vi "Fetch (Waveform).vi"(0 "VISA resource name":refnum<visa-resource-name>, 1 "Segment Index (0)":i32 format="%.0g", 5 "Measurement Source (1: Channel 1)":i32(ring)=1 items=["Channel 1"=1, "Channel 2"=2, "Channel 3"=3, "Channel 4"=4, "Function 1"=5, "Function 2"=6, "Function 3"=7, "Function 4"=8, "Memory 1"=9, "Memory 2"=10, "Memory 3"=11, "Memory 4"=12], 9 "Maximum Time (10000ms)":u32=10000, 11 "error in (no error)":errorcluster) -> (4 "VISA resource name out":refnum<visa-resource-name>, 8 "Waveform Data":waveform(dbl)(graph), 15 "error out":errorcluster)   [LabVIEW 2020, in "Agilent 90000 Series.lvlib"]
doc: "Returns the waveform the oscilloscope acquired for the specified channel. The waveform is from an acquisition that you initiate prior to calling this VI.\n\nYou use the Initiate VI to start an acquisition on the channels that you enable with the Configure Channel VI. The oscilloscope acquires waveforms for the enabled channels concurrently. You must call this VI separately for each enabled channel to obtain the waveforms.\n\nYou can call the Read Waveform VI instead of using low-level VIs.\n\n<B>Note:</B> Use this VI only with other low-level VIs. The high-level VIs automatically incorporate this functionality. This VI does not check the instrument status."
uses:
  Agilent 90000 Series.lvlib
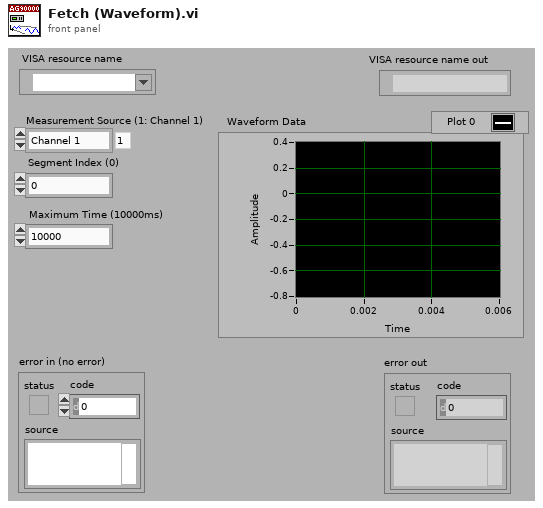
[diagram p1: front panel]
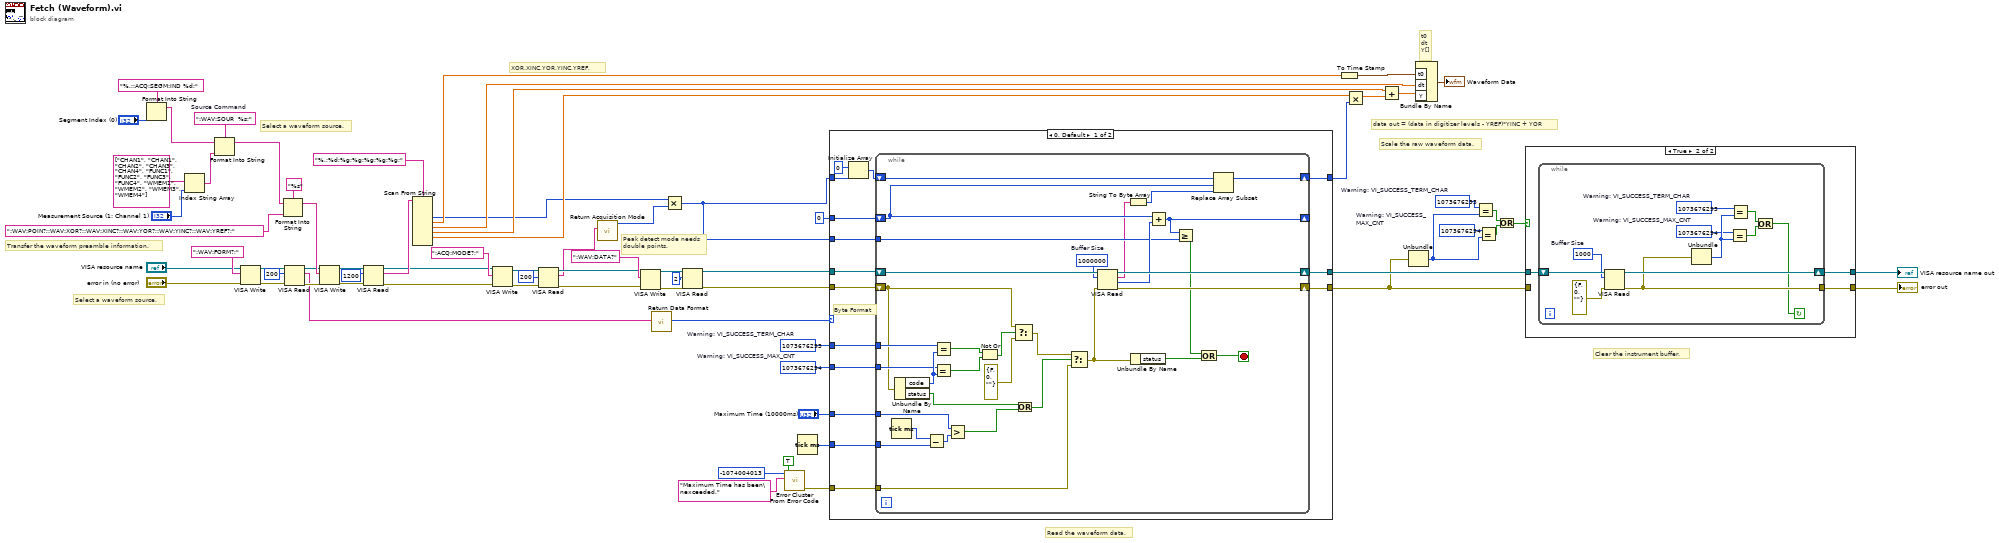
[diagram p0: block diagram]
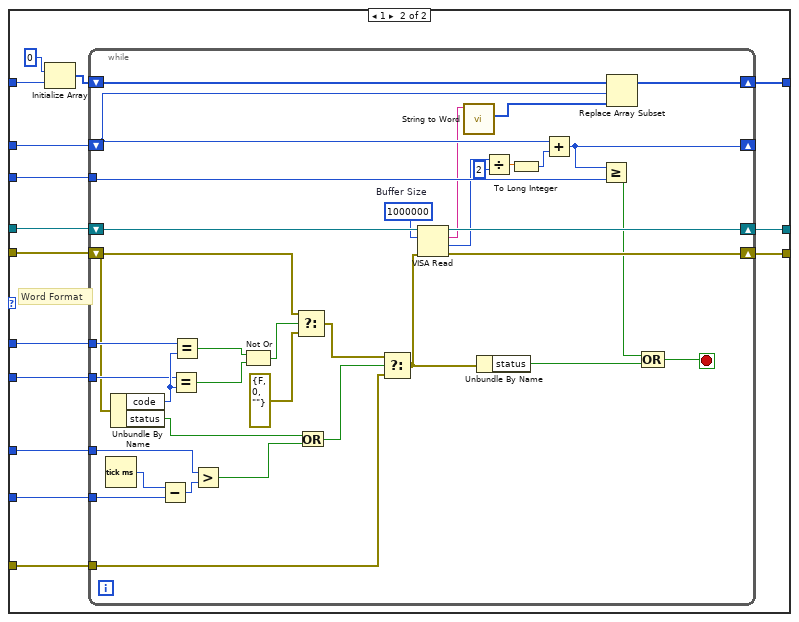
[diagram p2: hidden frame]
diagram:
  w49 = 1073676294  # Warning: VI_SUCCESS_MAX_CNT
  w48 = 1073676293  # Warning: VI_SUCCESS_TERM_CHAR
  w41 = 1073676294  # Warning: VI_SUCCESS_MAX_CNT
  w40 = 1073676293  # Warning: VI_SUCCESS_TERM_CHAR
  w67 = ":WAV:SOUR  %s;"  # Source Command
  # "Peak detect mode needs\ndouble points."
  # "Select a waveform source."
  # "Transfer the waveform preamble information."
  # "Scale the raw waveform data."
  # "Clear the instrument buffer."
  # "Read the waveform data."
  # "Select a waveform source."
  # "XOR,XINC,YOR,YINC,YREF,"
  # "data out = (data in digitizer levels - YREF)*YINC + YOR"
  # "t0\ndt\nY[]"
  n1 = Format Into String(format string="%.;:ACQ:SEGM:IND %d;", "Segment Index (0)") -> (resulting string=w56:string)  [unwired: 2 in, 1 out]
  n2 = Index String Array(1:"Measurement Source (1: Channel 1)", 2:string[] ["CHAN1", "CHAN1", "CHAN2", "CHAN3", "CHAN4", "FUNC1", "FUNC2", "FUNC3", "FUNC4", "WMEM1", "WMEM2", "WMEM3", "WMEM4"] ("subarray 2")) -> (0:w60:string)  [unwired: 1 out]
  n3 = Format Into String(format string=w67, initial string=w56, w60) -> (resulting string=w65:string)  [unwired: 1 in, 1 out]
  n4 = VISA Write(VISA resource name="VISA resource name", write buffer=":WAV:FORM?;", error in (no error)="error in (no error)") -> (VISA resource name out=w22:refnum<visa-resource-name>, error out=w21:errorcluster)  [unwired: 1 out]
  n5 = Format Into String(format string="%s", initial string=w65, ":WAV:POIN?;:WAV:XOR?;:WAV:XINC?;:WAV:YOR?;:WAV:YINC?;:WAV:YREF?;") -> (resulting string=w64:string)  [unwired: 1 in, 1 out]
  n6 = VISA Read(VISA resource name=w22, byte count=u32 200, error in (no error)=w21) -> (VISA resource name out=w18:refnum<visa-resource-name>, read buffer=w16:string, error out=w17:errorcluster)  [unwired: 1 out]
  n7 = VISA Write(VISA resource name=w18, write buffer=w64, error in (no error)=w17) -> (VISA resource name out=w72:refnum<visa-resource-name>, error out=w71:errorcluster)  [unwired: 1 out]
  n8 = VISA Read(VISA resource name=w72, byte count=u32 1200, error in (no error)=w71) -> (VISA resource name out=w5:refnum<visa-resource-name>, read buffer=w24:string, error out=w4:errorcluster)  [unwired: 1 out]
  n9 = Scan From String(format string="%.;%d;%g;%g;%g;%g;%g;", input string=w24) -> (output 1=w9:i32, output 2=w13:dbl, output 3=w12:dbl, output 4=w11:dbl, output 5=w10:dbl)  [unwired: 2 in, 10 out]
  n10 = VISA Write(VISA resource name=w5, write buffer=":ACQ:MODE?;", error in (no error)=w4) -> (VISA resource name out=w29:refnum<visa-resource-name>, error out=w28:errorcluster)  [unwired: 1 out]
  n11 = VISA Read(VISA resource name=w29, byte count=u32 200, error in (no error)=w28) -> (VISA resource name out=w27:refnum<visa-resource-name>, read buffer=w1:string, error out=w26:errorcluster)  [unwired: 1 out]
  n12 = call "Return Acquisition Mode.vi"("Acquisition Mode"=w1) -> ("Multiply Factor"=w2:i32)  [unwired: 10 out]
  n13 = VISA Write(VISA resource name=w27, write buffer=":WAV:DATA?", error in (no error)=w26) -> (VISA resource name out=w37:refnum<visa-resource-name>, error out=w36:errorcluster)  [unwired: 1 out]
  n14 = call "Return Data Format.vi"("String In"=w16) -> ("Data Format"=w3:u16)  [unwired: 10 out]
  n15 = Multiply(x=w9, y=w2) -> (x*y=w8:i32)
  n16 = VISA Read(VISA resource name=w37, byte count=u32 2, error in (no error)=w36) -> (VISA resource name out=w7:refnum<visa-resource-name>, error out=w6:errorcluster)  [unwired: 2 out]
  n17 = call <vilib>:"Error Cluster From Error Code.vi"("show call chain? (False)"=TRUE, "error message (\"\")"="Maximum Time has been\nexceeded." ("error message (\"\")"), "error code (0)"=-1074004013) -> ("error out"=w47:errorcluster)  [unwired: 1 in, 5 out]
  n18 = Tick Count (ms)() -> (millisecond timer value=w46:u32)
  n19 = case shown="0, Default" w3 {
    tunnel: [w87 w135] -> w55
    tunnel: [w86 w134] -> w54
    tunnel: w47 -> [w85 w133]
    tunnel: w46 -> [w84 w132]
    tunnel: "Maximum Time (10000ms)" -> [w83 w131]
    tunnel: w41 -> [w82 w130]
    tunnel: w40 -> [w81 w129]
    tunnel: 0 ("index") -> [w80 w128]
    tunnel: w8 -> [w73 w122]
    tunnel: w7 -> [w79 w127]
    tunnel: [w78 w126] -> w32
    tunnel: w8 -> [w77 w125]
    tunnel: w6 -> [w76 w124]
    frame 0, Default {
      # "Byte Format"
      n20 = Initialize Array(i8 0 ("element"), w73) -> (w74:i8[])
      n21 = while {
        shift-right: [w115] -> w86
        shift-left: w76 -> [w102]
        shift-right: [w120] -> w87
        shift-left: w79 -> [w119]
        shift-right: [w116] -> w78
        shift-left: w74 -> [w117]
        shift-right: [w112] -> _
        shift-left: w80 -> [w113]
        tunnel: w77 -> [w111]
        tunnel: w81 -> [w104]
        tunnel: w82 -> [w103]
        tunnel: w83 -> [w99]
        tunnel: w84 -> [w98]
        tunnel: w85 -> [w93]
        stop <- w90 stop-if-true
        w118 = u32 1000000  # Buffer Size
        n22 = Tick Count (ms)() -> (millisecond timer value=w100:u32)
        n23 = Unbundle By Name(w102) -> ("code"=w105:i32, "status"=w97:bool)
        n24 = Subtract(x=w100, y=w98) -> (x-y=w101:u32)
        n25 = Equal?(x=w103, y=w105) -> (x = y?=w108:bool)
        n26 = Equal?(x=w104, y=w105) -> (x = y?=w109:bool)
        n27 = Greater?(x=w99, y=w101) -> (0:w96:bool)
        n28 = Not Or(1:w108, 2:w109) -> (0:w107:bool)
        n29 = Select(t=w102, s=w107, f=errorcluster {"status"=FALSE, "code"=0, "source"=""} ("error in (no error)")) -> (s? t:f=w95:errorcluster)
        n30 = Or(x=w97, y=w96) -> (x .or. y?=w94:bool)
        n31 = Select(t=w95, s=w94, f=w93) -> (s? t:f=w92:errorcluster)
        n32 = VISA Read(VISA resource name=w119, byte count=w118, error in (no error)=w92) -> (VISA resource name out=w120:refnum<visa-resource-name>, read buffer=w89:string, return count=w114:u32, error out=w115:errorcluster)
        n33 = String To Byte Array(string=w89) -> (unsigned byte array=w88:u8[])
        n34 = Unbundle By Name(w92) -> ("status"=w91:bool)
        n35 = Add(x=w113, y=w114) -> (x+y=w112:u32)
        n36 = Greater Or Equal?(x=w112, y=w111) -> (x >= y?=w110:bool)
        n37 = Compound Arithmetic op=OR(w110, w91) -> (w90:bool)
        n38 = Replace Array Subset(array=w117, new element=w88, index=w113) -> (w116:i8[])
      }
    }
    frame 1 {
      # "Word Format"
      n39 = Initialize Array(i16 0 ("element"), w122) -> (w121:i16[])
      n40 = while {
        shift-right: [w166] -> w134
        shift-left: w124 -> [w154]
        shift-right: [w171] -> w135
        shift-left: w127 -> [w170]
        shift-right: [w167] -> w126
        shift-left: w121 -> [w168]
        shift-right: [w164] -> _
        shift-left: w128 -> [w165]
        tunnel: w125 -> [w163]
        tunnel: w129 -> [w156]
        tunnel: w130 -> [w155]
        tunnel: w131 -> [w151]
        tunnel: w132 -> [w150]
        tunnel: w133 -> [w145]
        stop <- w142 stop-if-true
        w169 = u32 1000000  # Buffer Size
        n41 = Tick Count (ms)() -> (millisecond timer value=w152:u32)
        n42 = Unbundle By Name(w154) -> ("code"=w157:i32, "status"=w149:bool)
        n43 = Subtract(x=w152, y=w150) -> (x-y=w153:u32)
        n44 = Equal?(x=w155, y=w157) -> (x = y?=w160:bool)
        n45 = Equal?(x=w156, y=w157) -> (x = y?=w161:bool)
        n46 = Greater?(x=w151, y=w153) -> (0:w148:bool)
        n47 = Not Or(1:w160, 2:w161) -> (0:w159:bool)
        n48 = Select(t=w154, s=w159, f=errorcluster {"status"=FALSE, "code"=0, "source"=""} ("error in (no error)")) -> (s? t:f=w147:errorcluster)
        n49 = Or(x=w149, y=w148) -> (x .or. y?=w146:bool)
        n50 = Select(t=w147, s=w146, f=w145) -> (s? t:f=w144:errorcluster)
        n51 = VISA Read(VISA resource name=w170, byte count=w169, error in (no error)=w144) -> (VISA resource name out=w171:refnum<visa-resource-name>, read buffer=w141:string, return count=w138:u32, error out=w166:errorcluster)
        n52 = call "String to Word.vi"("String"=w141) -> ("Int16 Data"=w140:i16[])  [unwired: 1 in, 9 out]
        n53 = Unbundle By Name(w144) -> ("status"=w143:bool)
        n54 = Divide(x=w138, y=u32 2) -> (x/y=w136:dbl)
        n55 = To Long Integer(number=w136) -> (32bit integer=w139:i32)
        n56 = Add(x=w165, y=w139) -> (x+y=w164:i32)
        n57 = Greater Or Equal?(x=w164, y=w163) -> (x >= y?=w162:bool)
        n58 = Replace Array Subset(array=w168, new element=w140, index=w165) -> (w167:i16[])
        n59 = Compound Arithmetic op=OR(w162, w143) -> (w142:bool)
      }
    }
  }
  n60 = To Time Stamp(1:w13) -> (0:w69:timestamp)
  n61 = Multiply(x=w10, y=w32) -> (x*y=w62:dbl[])
  n62 = Add(x=w11, y=w62) -> (x+y=w63:dbl[])
  n63 = Unbundle(w54) -> ("code"=w50:i32)  [unwired: 2 out]
  n64 = Bundle By Name ("Build Waveform")("t0"=w69, "dt"=w12, "Y"=w63) -> (→"Waveform Data":waveform(dbl))  [unwired: 1 out]
  n65 = Equal?(x=w48, y=w50) -> (x = y?=w53:bool)
  n66 = Equal?(x=w49, y=w50) -> (x = y?=w52:bool)
  n67 = Or(x=w53, y=w52) -> (x .or. y?=w51:bool)
  n68 = case shown="True" w51 {
    tunnel: w55 -> [w173 w176]
    tunnel: w54 -> [w172 _]
    tunnel: [w173 w175] -> w34
    tunnel: [w172 w174] -> w33
    frame False {
    }
    frame True {
      n69 = while {
        shift-right: [w186] -> w175
        shift-left: w176 -> [w187]
        tunnel: [w179] -> w174
        stop <- w178 continue-if-true
        w181 = 1073676294  # Warning: VI_SUCCESS_MAX_CNT
        w180 = 1073676293  # Warning: VI_SUCCESS_TERM_CHAR
        w185 = u32 1000  # Buffer Size
        n70 = VISA Read(VISA resource name=w187, byte count=w185, error in (no error)=errorcluster {"status"=FALSE, "code"=0, "source"=""}) -> (VISA resource name out=w186:refnum<visa-resource-name>, error out=w179:errorcluster)  [unwired: 2 out]
        n71 = Unbundle(w179) -> ("code"=w182:i32)  [unwired: 2 out]
        n72 = Equal?(x=w181, y=w182) -> (x = y?=w183:bool)
        n73 = Equal?(x=w180, y=w182) -> (x = y?=w184:bool)
        n74 = Or(x=w184, y=w183) -> (x .or. y?=w178:bool)
      }
    }
  }
  "error out" <- w33
  "VISA resource name out" <- w34
